vi "snapPoint.vi"(0 "reference":refnum<class "Grid.lvclass">, 1 "point2D":T1 {"y" format="%.2f"; "x" format="%.2f"}, 5 "error in (no error)":errorcluster) -> (14 "reference out":refnum<class "Grid.lvclass">, 15 "point2D 2":T1 {"y" format="%.2f"; "x" format="%.2f"}, 19 "error out":errorcluster)   [LabVIEW 2012, in "Grid.lvclass"]
doc: "public void snap(Point2D p)"
uses:
  <resource>/Framework/Providers/Open_GDS/UML/Grid_class/Grid.lvclass
  <resource>/Framework/Providers/Open_GDS/UML/General/Point/Point Point2D.ctl
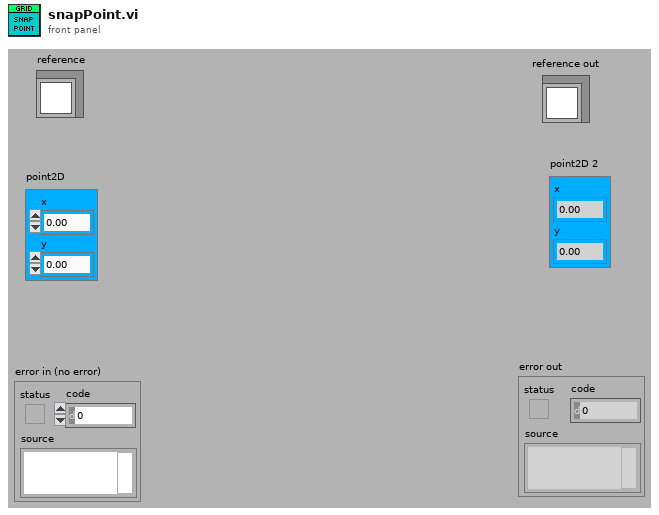
[diagram p1: front panel]
types:
  T1 = typedef "Point Point2D.ctl" = cluster{"x":dbl, "y":dbl}
  T2 = typedef "Grid.lvclass/ObjectAttributes.ctl" = cluster{"gridX":dbl, "gridY":dbl, "gridColor":u32}
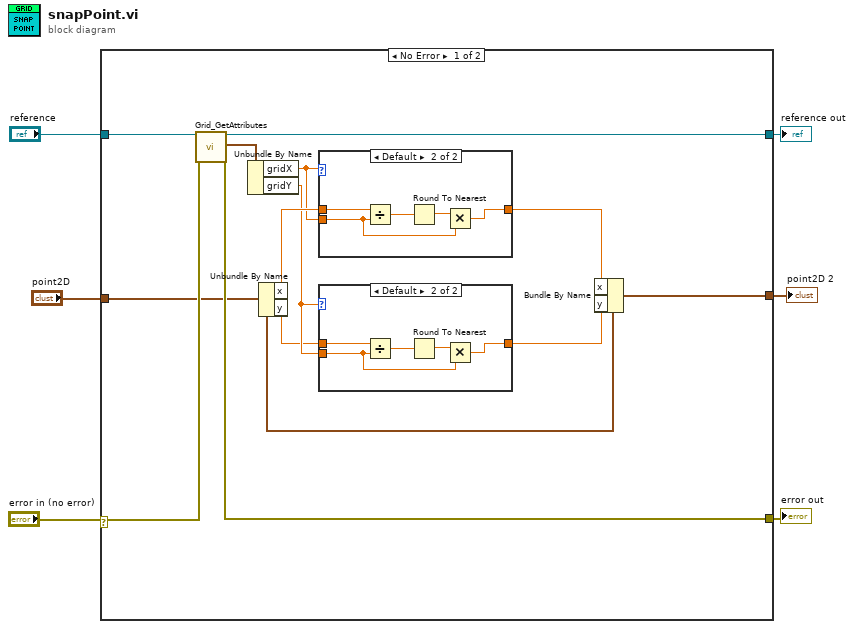
[diagram p0: block diagram]
diagram:
  n1 = case shown="No Error" "error in (no error)" {
    selector: "error in (no error)" -> [w15 w32]
    tunnel: "reference" -> [w19 w33]
    tunnel: [w18 w32] -> w5
    tunnel: [w17 w33] -> w4
    tunnel: "point2D" -> [w14 _]
    tunnel: [w13 _] -> w1
    frame No Error {
      n2 = call <resource>:"Grid_GetAttributes.vi"("reference in"=w19, "error in (no error)"=w15) -> ("reference out"=w17:refnum<class "Grid.lvclass">, "Attributes"=w16:T2, "error out"=w18:errorcluster)  [unwired: 15 out]
      n3 = Unbundle By Name(w16) -> ("gridX"=w11:dbl, "gridY"=w9:dbl)
      n4 = Unbundle By Name(w14) -> ("x"=w12:dbl, "y"=w8:dbl)
      n5 = case shown="Default" w11 {
        tunnel: w12 -> [w26 w31]
        tunnel: w11 -> [_ w28]
        tunnel: [w26 w27] -> w10
        frame 0 {
        }
        frame Default {
          n6 = Divide(x=w31, y=w28) -> (x/y=w30:dbl)
          n7 = Round To Nearest(number=w30) -> (nearest integer value=w29:dbl)
          n8 = Multiply(x=w29, y=w28) -> (x*y=w27:dbl)
        }
      }
      n9 = case shown="Default" w9 {
        tunnel: w8 -> [w20 w25]
        tunnel: w9 -> [_ w22]
        tunnel: [w20 w21] -> w7
        frame 0 {
        }
        frame Default {
          n10 = Divide(x=w25, y=w22) -> (x/y=w24:dbl)
          n11 = Round To Nearest(number=w24) -> (nearest integer value=w23:dbl)
          n12 = Multiply(x=w23, y=w22) -> (x*y=w21:dbl)
        }
      }
      n13 = Bundle By Name(cluster=w14, "x"=w10, "y"=w7) -> (w13:T1)
    }
    frame Error {
    }
  }
  "reference out" <- w4
  "error out" <- w5
  "point2D 2" <- w1
